vi "Write to Hardware.vi"(8 "error in":errorcluster, 9 "Trigger Values":dbl[](array[numeric]), 10 "Values":dbl[](array[numeric]), 11 "Tx Execution Unit Implementation in":refnum<class "Tx Execution Unit.lvclass">) -> (0 "error out":errorcluster, 1 "Trigger Values out":dbl[](array[numeric]), 2 "Values out":dbl[](array[numeric]), 3 "Tx Execution Unit Implementation out":refnum<class "Tx Execution Unit.lvclass">)   [LabVIEW 2020, in "Ballard MIL-STD-1553 Engine.lvlib" / "Implementation.lvlib" / "Tx Execution Unit.lvclass"]
uses:
  Tx Execution Unit.lvclass
  C:/Users/nitest/Desktop/Git 2020/niveristand-aim-milStd1553-custom-device/Source/Custom Device Support/Engine/Implementation/Execution Unit/Execution Unit.lvclass
  Execution Unit/Execution Unit.lvclass/Execution Unit.ctl
  Tx Execution Unit.lvclass/Tx Execution Unit.ctl
  AIM 1553 Examples/New Wrapped API/Module Reference.ctl
  <instrlib>/BTI1553Lib/BTI1553LV.lvlib
  Execution Unit/Execution Unit.lvclass
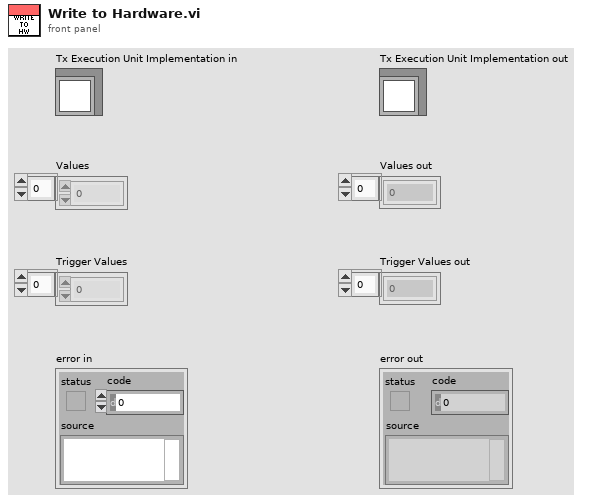
[diagram p1: front panel]
types:
  T1 = typedef "Ballard MIL-STD-1553 Engine.lvlib/Custom Device.lvlib/Hardware Handles.ctl" = cluster{"core handle":u64, "core reader handle":u64, "channel handles":u64[]}
  T2 = typedef "1553 Channel.ctl" = cluster{"HW channel":u16, "terminal addresses":T3[], "terminal names":string[], "acyclic frame names":string[], "messages":T4[]}
  T3 = typedef "Address.ctl" = u16
  T4 = typedef "Message Definition.ctl" = cluster{"name":string, "message type":T5, "endpoint Tx":T6, "endpoint Rx":T6, "create timestamp channel":bool, "mode code":u16, "number of words":u16, "parameters":cluster{"name":string, "default value":dbl, "unit":string, "parameter definition":T7}[]}
  T5 = typedef "Message Type.ctl" = string
  T6 = typedef "Terminal Endpoint.ctl" = cluster{"terminal address":T3, "subaddress":T3}
  T7 = typedef "Parameter Definition.ctl" = cluster{"start index":i32, "size (bits)":i32, "encoding":enum16{"BNR", "BCD", "Discrete"}, "signed":bool, "multiplier":dbl, "offset":dbl}
  T8 = typedef "Map of Message Indexes to Tx Write Info.ctl" = map{i32, T9}
  T9 = typedef "Tx Write Info.ctl" = cluster{"transfer handle":u64, "value index":i32}
  T10 = typedef "Module Reference.ctl" = cluster{"Module Handle":u32, "BIU Number":u8}
  T11 = enum16{"unknown", "BC Message Buffer", "RT Message Buffer"}
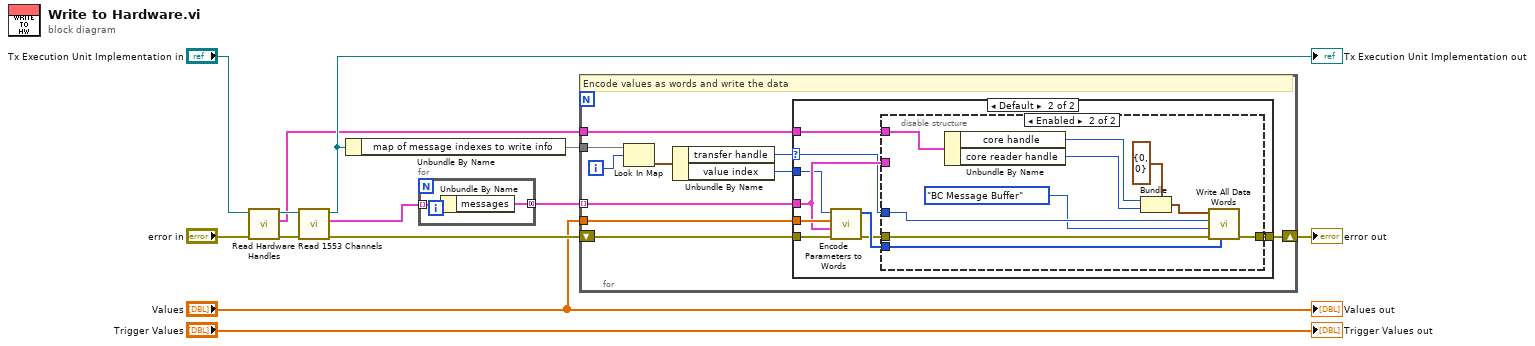
[diagram p0: block diagram]
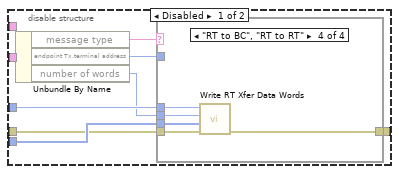
[diagram p3: hidden frame]
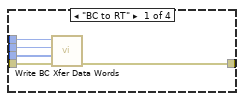
[diagram p4: hidden frame]
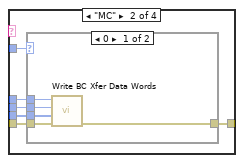
[diagram p5: hidden frame]
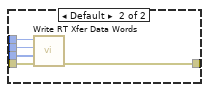
[diagram p6: hidden frame]
diagram:
  n1 = call "Read Hardware Handles.vi"("error in"="error in", "Execution Unit in"="Tx Execution Unit Implementation in") -> ("error out"=w2:errorcluster, "hardware handles"=w1:T1, "Execution Unit out"=w3:refnum<class "Tx Execution Unit.lvclass">)  [unwired: 7 in]
  n2 = call "Read 1553 Channels.vi"("error in"=w2, "Execution Unit in"=w3) -> ("error out"=w9:errorcluster, "1553 channels"=w10:T2[], "Execution Unit out"=w6:refnum<class "Tx Execution Unit.lvclass">)  [unwired: 7 in]
  "Tx Execution Unit Implementation out" <- w6
  n3 = Unbundle By Name(w6) -> ("map of message indexes to write info"=w11:T8)
  n4 = for {
    tunnel: w10 -> [w14] mode=indexing
    tunnel: [w15] -> w8 mode=concatenating
    n5 = Unbundle By Name(w14) -> ("messages"=w15:T4[])
  }
  n6 = for {
    shift-right: [w25] -> w12
    shift-left: w9 -> [w21]
    tunnel: w11 -> [w24]
    tunnel: w8 -> [w19] mode=indexing
    tunnel: "Values" -> [w20]
    tunnel: w1 -> [w16]
    i -> [w23]
    # "Encode values as words and write the data"
    n7 = Look In Map(map=w24, key=w23) -> (value=w22:T9)  [unwired: 1 in, 1 out]
    n8 = Unbundle By Name(w22) -> ("transfer handle"=w18:u64, "value index"=w17:i32)
    n9 = case shown="Default" w18 {
      selector: w18 -> [_ w33]
      tunnel: w20 -> [_ w35]
      tunnel: w19 -> [_ w34]
      tunnel: w17 -> [_ w32]
      tunnel: [w26 w30] -> w25
      tunnel: w21 -> [w26 w29]
      tunnel: w16 -> [_ w27]
      frame 0, -1 {
      }
      frame Default {
        n10 = call "Encode Parameters to Words.vi"("error in"=w29, "message"=w34, "Values"=w35, "value index"=w32) -> ("error out"=w28:errorcluster, "data words"=w31:u16[])  [unwired: 6 in]
        n11 = disable-structure shown="Enabled" {
          disable-tunnel: w34 -> [w43 _]
          disable-tunnel: w33 -> [w42 w79]
          disable-tunnel: w31 -> [w40 w77]
          disable-tunnel: [w38 w76] -> w30
          disable-tunnel: w28 -> [w37 w80]
          disable-tunnel: w27 -> [_ w71]
          frame Disabled {
            n12 = Unbundle By Name(w43) -> ("message type"=w36:T5, "endpoint Tx.terminal address"=w39:T3, "number of words"=w41:u16)
            n13 = case shown="\"RT to BC\", \"RT to RT\"" w36 {
              tunnel: [w44 w50 w65 w70] -> w38
              tunnel: w41 -> [w46 w52 _ w69]
              tunnel: w42 -> [w45 w51 _ w68]
              tunnel: w40 -> [w47 w53 _ w67]
              tunnel: w37 -> [w48 w54 w65 w66]
              tunnel: w39 -> [_ w49 _ _]
              frame "BC to RT" {
                n14 = call <instrlib>:"Write BC Xfer Data Words.vi"("error in (no error)"=w48, "data words"=w47, "data word count in"=w46, "bc transfer handle in"=w45) -> ("error out"=w44:errorcluster)  [unwired: 5 in, 2 out]
              }
              frame "MC" {
                n15 = case shown="0" w49 {
                  tunnel: w54 -> [w59 w64]
                  tunnel: w53 -> [w58 w60]
                  tunnel: w52 -> [w57 w61]
                  tunnel: w51 -> [w56 w62]
                  tunnel: [w55 w63] -> w50
                  frame 0 {
                    n16 = call <instrlib>:"Write BC Xfer Data Words.vi"("error in (no error)"=w59, "data words"=w58, "data word count in"=w57, "bc transfer handle in"=w56) -> ("error out"=w55:errorcluster)  [unwired: 5 in, 2 out]
                  }
                  frame Default {
                    n17 = call <instrlib>:"Write RT Xfer Data Words.vi"("error in (no error)"=w64, "data words"=w60, "data word count in"=w61, "rt transfer handle in"=w62) -> ("error out"=w63:errorcluster)  [unwired: 5 in, 2 out]
                  }
                }
              }
              frame Default {
              }
              frame "RT to BC", "RT to RT" {
                n18 = call <instrlib>:"Write RT Xfer Data Words.vi"("error in (no error)"=w66, "data words"=w67, "data word count in"=w69, "rt transfer handle in"=w68) -> ("error out"=w70:errorcluster)  [unwired: 5 in, 2 out]
              }
            }
          }
          frame Enabled {
            n19 = Unbundle By Name(w71) -> ("core handle"=w74:u64, "core reader handle"=w73:u64)
            n20 = Bundle(cluster=T10 {"Module Handle"=0, "BIU Number"=0} ("Module Reference"), "Module Handle"=w74, "BIU Number"=w73) -> (w72:T10)
            n21 = call "Write All Data Words.vi"("Data Words"=w77, "Error In"=w80, "Buffer Type"=T11."BC Message Buffer" ("Buffer Type (BC)"), "Buffer Header and Buffer ID"=w79, "Module Reference"=w72) -> ("Error Out"=w76:errorcluster)  [unwired: 5 in, 1 out]
          }
        }
      }
    }
  }
  "error out" <- w12
  "Values out" <- "Values"
  "Trigger Values out" <- "Trigger Values"
